vi "Remove Rows.vi"(4 "Rows":i32[](array[numeric]), 6 "Mode":enum16{"Selected Rows", "Input Rows"}(ring), 8 "error in (no error)":errorcluster, 11 "DataGridView in":refnum<class "DataGridView.lvclass">) -> (0 "error out":errorcluster, 3 "DataGridView out":refnum<class "DataGridView.lvclass">)   [LabVIEW 2016, in "DataGrid.lvlib" / "DataGridView.lvclass"]
doc: "This VI allows you to remove rows from the data table. The mode input chooses if you are removing specific rows or selected rows."
uses:
  <userlib>/LabVIEWdotNetDataGrid/source/DataGridView/DataGridView.lvclass
  <userlib>/LabVIEWdotNetDataGrid/source/DataGridView/DataGridView.lvclass/DataGridView.ctl
  System.Windows.Forms
  <userlib>/LabVIEWdotNetDataGrid/source/DataTable/DataTable.lvclass/DataTable.ctl
  System.Data
  <userlib>/LabVIEWdotNetDataGrid/source/DataGridView/Properties/Read DataGridView.vi
  <userlib>/LabVIEWdotNetDataGrid/source/DataGridView/Properties/Read SelectionMode.vi
  <userlib>/LabVIEWdotNetDataGrid/source/DataTable/Read DataTable.vi
  <userlib>/LabVIEWdotNetDataGrid/source/DataTable/DataTable.lvclass
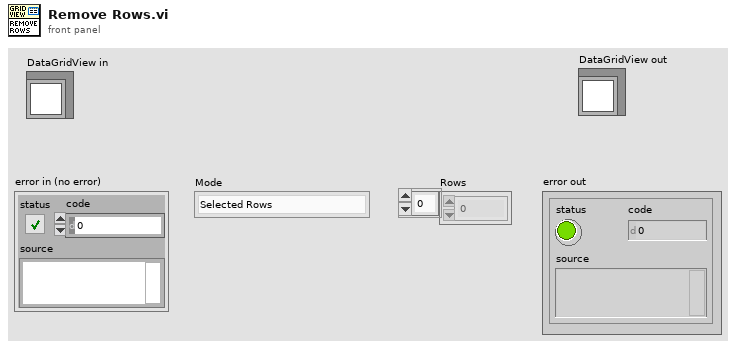
[diagram p1: front panel]
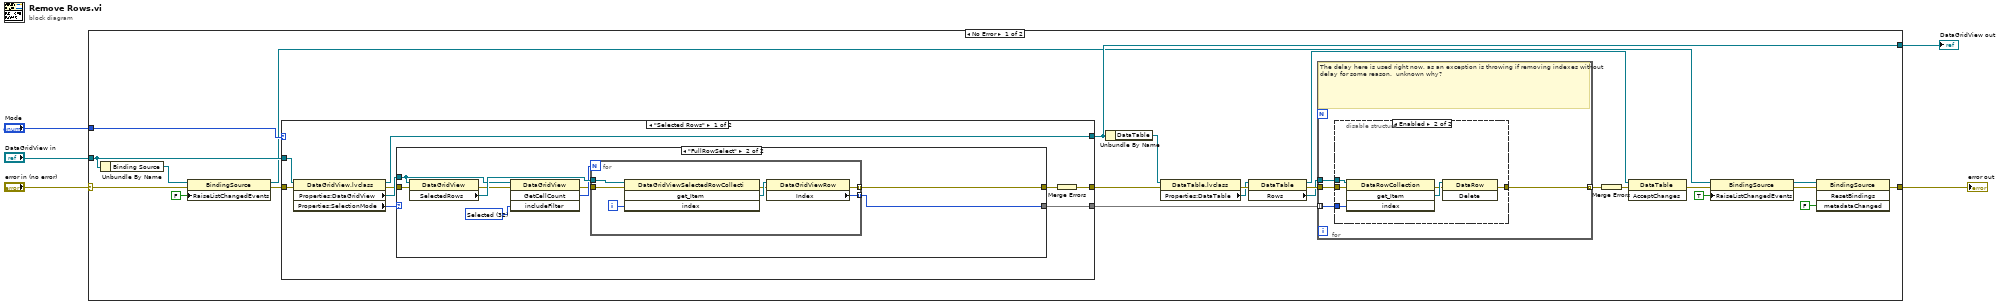
[diagram p0: block diagram]
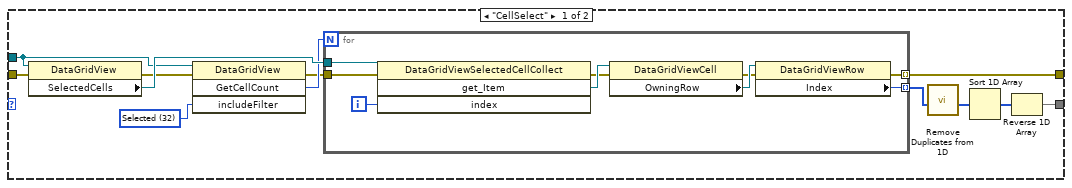
[diagram p2: hidden frame]
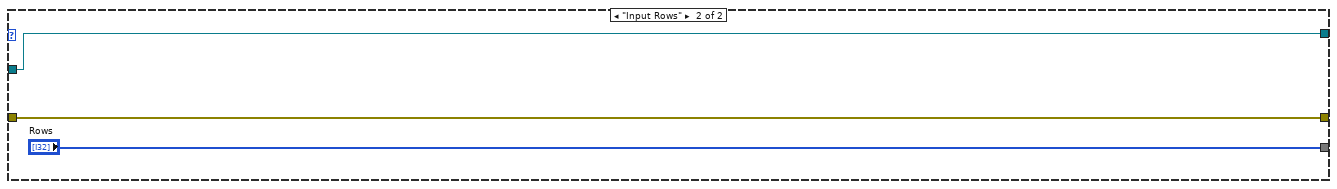
[diagram p3: hidden frame]
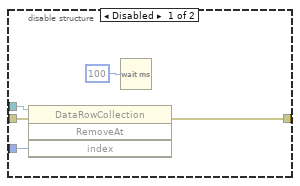
[diagram p4: hidden frame]
diagram:
  n1 = case shown="No Error" "error in (no error)" {
    selector: "error in (no error)" -> [w18 w95]
    tunnel: "DataGridView in" -> [w21 w94]
    tunnel: "Mode" -> [w26 _]
    tunnel: [w10 w95] -> w2
    tunnel: [w22 w94] -> w1
    frame No Error {
      n2 = Unbundle By Name(w21) -> ("Binding Source"=w19:refnum<k24>)
      n3 = property class="BindingSource"(reference=w19, error in=w18, "RaiseListChangedEvents"=FALSE) -> (reference out=w11:refnum<k24>, error out=w17:errorcluster)
      n4 = case shown="\"Selected Rows\"" w26 {
        tunnel: w21 -> [w38 w76]
        tunnel: [w31 w77] -> w25
        tunnel: [w36 "Rows"] -> w24
        tunnel: w17 -> [w32 w77]
        tunnel: [w30 w76] -> w22
        frame "Selected Rows" {
          n5 = property class="DataGridView.lvclass"(reference=w38, error in=w32) -> (reference out=w30:refnum<class "DataGridView.lvclass">, error out=w34:errorcluster, "Properties:DataGridView"=w35:refnum<k24>, "Properties:SelectionMode"=w33:enum16{"CellSelect", "FullRowSelect"})
          n6 = case shown="\"FullRowSelect\"" w33 {
            tunnel: [w49 w67] -> w37
            tunnel: [w41 w66] -> w36
            tunnel: w35 -> [w48 w65]
            tunnel: w34 -> [w43 w60]
            frame "CellSelect" {
              w47 = 32 items=["None"=0, "Displayed"=1, "Frozen"=2, "ReadOnly"=4, "Resizable"=8, "ResizableSet"=16, "Selected"=32, "Visible"=64] ("includeFilter")
              n7 = property class="DataGridView"(reference=w48, error in=w43) -> (error out=w45:errorcluster, "SelectedCells"=w50:refnum<k24>)  [unwired: 1 out]
              n8 = invoke class="DataGridView" method="GetCellCount"(reference=w48, error in=w45, "includeFilter"=w47) -> (error out=w44:errorcluster, "GetCellCount"=w46:i32)  [unwired: 1 in, 2 out]
              n9 = for {
                N: w46 -> [_]
                tunnel: w50 -> [w56]
                tunnel: [w54] -> w40 mode=indexing
                tunnel: [w52] -> w49 mode=indexing
                tunnel: w44 -> [w51]
                i -> [w58]
                n10 = invoke class="DataGridViewSelectedCellCollect" method="get_Item"(reference=w56, error in=w51, "index"=w58) -> (error out=w57:errorcluster, "get_Item"=w59:refnum<k24>)  [unwired: 1 in, 2 out]
                n11 = property class="DataGridViewCell"(reference=w59, error in=w57) -> (error out=w53:errorcluster, "OwningRow"=w55:refnum<k24>)  [unwired: 1 out]
                n12 = property class="DataGridViewRow"(reference=w55, error in=w53) -> (error out=w52:errorcluster, "Index"=w54:i32)  [unwired: 1 out]
              }
              n13 = call <userlib>:"Remove Duplicates from 1D.vi"("Input Array"=w40) -> ("No Duplicates Array"=w39:i32[])  [unwired: 10 in]
              n14 = Sort 1D Array(array=w39) -> (sorted array=w42:i32[])
              n15 = Reverse 1D Array(array=w42) -> (reversed array=w41:i32[])
            }
            frame "FullRowSelect" {
              w64 = 32 items=["None"=0, "Displayed"=1, "Frozen"=2, "ReadOnly"=4, "Resizable"=8, "ResizableSet"=16, "Selected"=32, "Visible"=64] ("includeFilter")
              n16 = property class="DataGridView"(reference=w65, error in=w60) -> (error out=w62:errorcluster, "SelectedRows"=w68:refnum<k24>)  [unwired: 1 out]
              n17 = invoke class="DataGridView" method="GetCellCount"(reference=w65, error in=w62, "includeFilter"=w64) -> (error out=w61:errorcluster, "GetCellCount"=w63:i32)  [unwired: 1 in, 2 out]
              n18 = for {
                N: w63 -> [_]
                tunnel: w68 -> [w74]
                tunnel: [w73] -> w66 mode=indexing
                tunnel: [w72] -> w67 mode=indexing
                tunnel: w61 -> [w71]
                i -> [w75]
                n19 = invoke class="DataGridViewSelectedRowCollecti" method="get_Item"(reference=w74, error in=w71, "index"=w75) -> (error out=w69:errorcluster, "get_Item"=w70:refnum<k24>)  [unwired: 1 in, 2 out]
                n20 = property class="DataGridViewRow"(reference=w70, error in=w69) -> (error out=w72:errorcluster, "Index"=w73:i32)  [unwired: 1 out]
              }
            }
          }
          n21 = Merge Errors(w37) -> (w31:errorcluster)
        }
        frame "Input Rows" {
        }
      }
      n22 = Unbundle By Name(w22) -> ("DataTable"=w23:refnum<class "DataTable.lvclass">)
      n23 = property class="DataTable.lvclass"(reference=w23, error in=w25) -> (error out=w29:errorcluster, "Properties:DataTable"=w9:refnum<k24>)  [unwired: 1 out]
      n24 = property class="DataTable"(reference=w9, error in=w29) -> (reference out=w6:refnum<k24>, error out=w28:errorcluster, "Rows"=w8:refnum<k24>)
      n25 = for {
        tunnel: w8 -> [w79]
        tunnel: w24 -> [w80] mode=indexing
        tunnel: w28 -> [w82]
        tunnel: [w81] -> w27 mode=indexing
        # "The delay here is used right now, as an exception is throwing if removing indexes without delay for some reason.  unknown why?"
        n26 = disable-structure shown="Enabled" {
          disable-tunnel: w82 -> [w87 w92]
          disable-tunnel: [w86 w88] -> w81
          disable-tunnel: w80 -> [w85 w91]
          disable-tunnel: w79 -> [w84 w93]
          frame Disabled {
            n27 = invoke class="DataRowCollection" method="RemoveAt"(reference=w84, error in=w87, "index"=w85) -> (error out=w86:errorcluster)  [unwired: 1 in, 3 out]
            n28 = Wait (ms)(milliseconds to wait=u32 100) -> ()  [unwired: 1 out]
          }
          frame Enabled {
            n29 = invoke class="DataRowCollection" method="get_Item"(reference=w93, error in=w92, "index"=w91) -> (error out=w89:errorcluster, "get_Item"=w90:refnum<k24>)  [unwired: 1 in, 2 out]
            n30 = invoke class="DataRow" method="Delete"(reference=w90, error in=w89) -> (error out=w88:errorcluster)  [unwired: 1 in, 2 out]
          }
        }
      }
      n31 = Merge Errors(w27) -> (w15:errorcluster)
      n32 = invoke class="DataTable" method="AcceptChanges"(reference=w6, error in=w15) -> (error out=w7:errorcluster)  [unwired: 1 in, 2 out]
      n33 = property class="BindingSource"(reference=w11, error in=w7, "RaiseListChangedEvents"=TRUE) -> (reference out=w12:refnum<k24>, error out=w13:errorcluster)
      n34 = invoke class="BindingSource" method="ResetBindings"(reference=w12, error in=w13, "metadataChanged"=FALSE) -> (error out=w10:errorcluster)  [unwired: 1 in, 3 out]
    }
    frame Error {
    }
  }
  "error out" <- w2
  "DataGridView out" <- w1
